vi "D Term.vi"(7 "Output Range":T1={"Min"=-50.0, "Max"=50.0}, 8 "Error":dbl=20.0, 9 "D Gain":dbl=0.5, 10 "Last Error":dbl=20.0, 11 "dT":dbl=0.1) -> (2 "Output":dbl)   [LabVIEW 2020, in "IG PID.lvlib" / "PID.lvclass"]
uses:
  PID.lvclass
  Output Range.ctl
  IG PID.lvlib
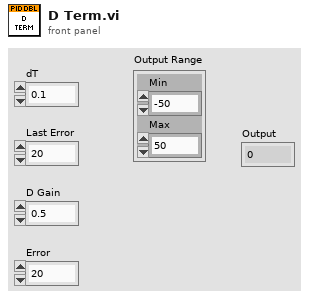
[diagram p1: front panel]
types:
  T1 = typedef "IG PID.lvlib/Output Range.ctl" = cluster{"Min":dbl, "Max":dbl}
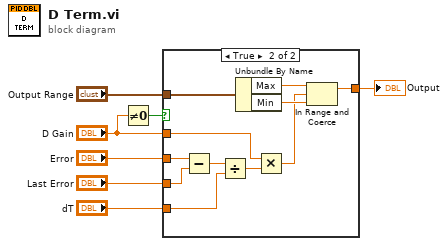
[diagram p0: block diagram]
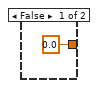
[diagram p2: hidden frame]
diagram:
  n1 = Not Equal To 0?(x="D Gain") -> (x != 0?=w1:bool)
  n2 = case shown="True" w1 {
    tunnel: "Output Range" -> [_ w19]
    tunnel: "Error" -> [_ w18]
    tunnel: "Last Error" -> [_ w17]
    tunnel: "dT" -> [_ w15]
    tunnel: [0.0 ("Max") w10] -> w3
    tunnel: "D Gain" -> [_ w9]
    frame False {
    }
    frame True {
      n3 = Subtract(x=w18, y=w17) -> (x-y=w16:dbl)
      n4 = Divide(x=w16, y=w15) -> (x/y=w14:dbl)
      n5 = Unbundle By Name(w19) -> ("Max"=w13:dbl, "Min"=w12:dbl)
      n6 = Multiply(x=w9, y=w14) -> (x*y=w11:dbl)
      n7 = In Range and Coerce(upper limit=w13, x=w11, lower limit=w12) -> (coerced(x)=w10:dbl)  [unwired: 1 out]
    }
  }
  "Output" <- w3
